vi "WSVCAP SHL Host LL RFFE Read.vi"(0 "RFFE Data [DUT Ordered]":u8[][](array[numeric]) format="%02x", 1 "Wait Ticks":u32, 2 "Slave Address":u8, 5 "Bytes to Read":u8, 7 "Socket Mask [U64]":u64=1 format="%02x", 11 "error in":errorcluster, 14 "FPGA":T1) -> (4 "RFFE Read Data [DUT Ordered]":u8[][](array[numeric]), 8 "Status":u8[](array[numeric]), 15 "error out":errorcluster)   [LabVIEW 2017]
uses:
  Type Defs/WSVCAP SHL FPGA Enum.ctl
  Type Defs/WSVCAP SHL Top Level Write Read State Enum.ctl
  Type Defs/WSVCAP SHL State.ctl
  Type Defs/WSVCAP SHL Top Level Control Enum.ctl
  Type Defs/WSVCAP SHL Transaction Enum.ctl
panel:
  out "Write Data":u64[](array[numeric]) format="%032b"
  out "Bit Array":u64[](array[numeric]) format="%.0x"
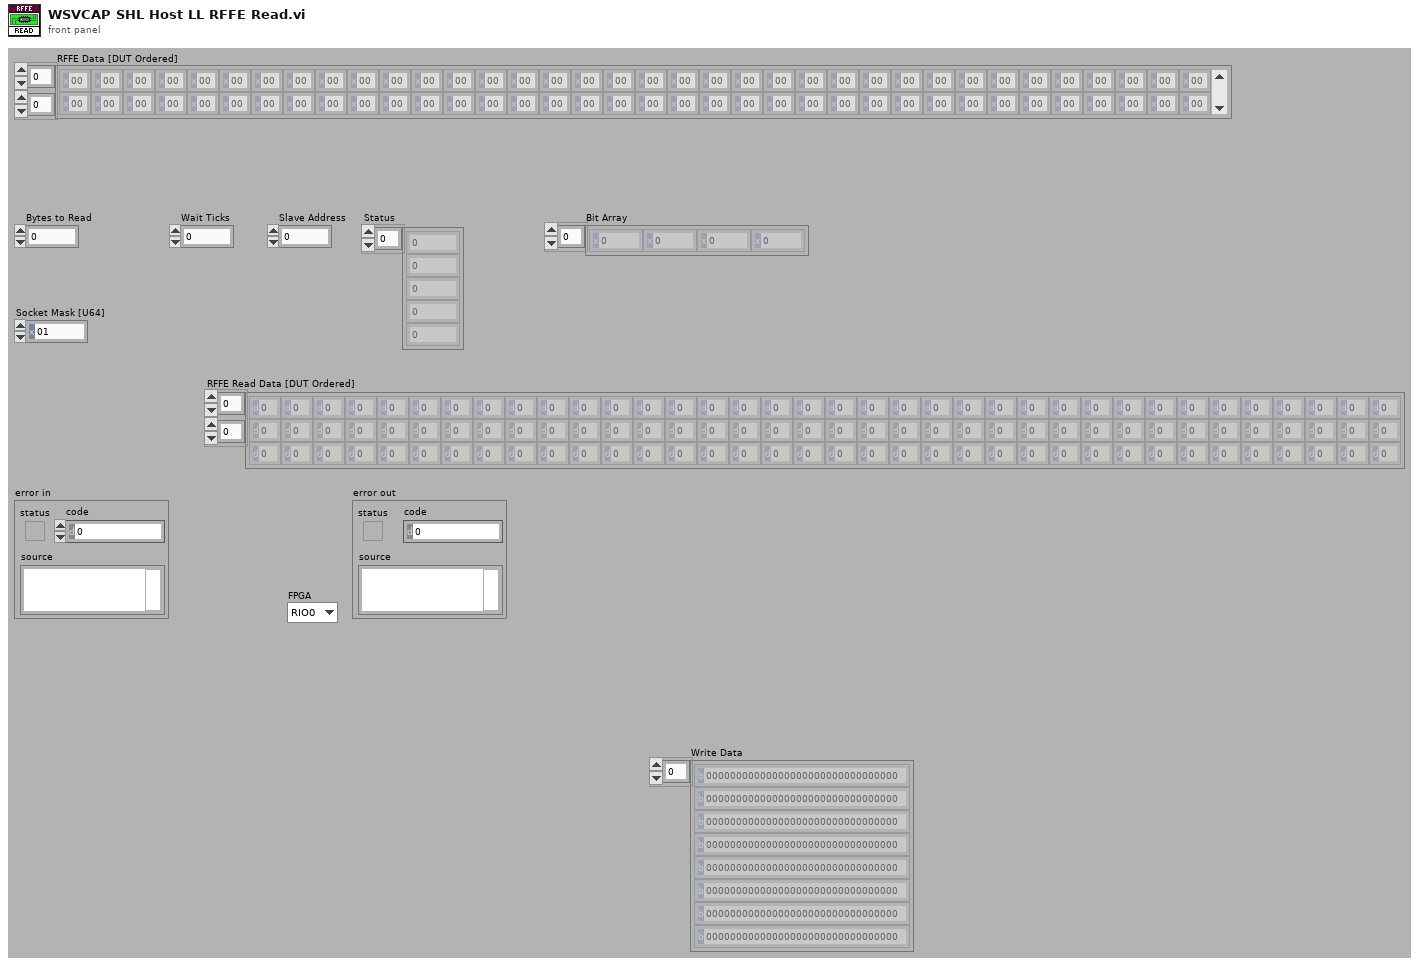
[diagram p1: front panel]
types:
  T1 = typedef "WSVCAP SHL FPGA Enum.ctl" = enum16{"RIO0", "RIO1"}
  T2 = typedef "WSVCAP SHL Top Level Write Read State Enum.ctl" = enum16{"Start", "Write", "Read", "Get Status", "Wait Until Done"}
  T3 = typedef "WSVCAP SHL State.ctl" = enum8{"Idle", "Transfer Data"}
  T4 = typedef "WSVCAP SHL Transaction Enum.ctl" = enum16{"I2C-Read Data", "I2C-Write Data", "RFFE-Ext Write", "RFFE-Ext Read"}
  T5 = typedef "WSVCAP SHL Top Level Control Enum.ctl" = enum16{"Start", "Cmd", "Transaction", "Wait Ticks", "Socket Mask", "UUT Set", "Slave Address", "Sub Address", "Bytes to Write", "Bytes to Read", "Write Data", "Write Flag", "Read Data", "Read Flag", "Ack Read", "Read Status Flag", "Ack Read Status", "Status", "Cycle Count", "Stop Cycle", "Exit"}
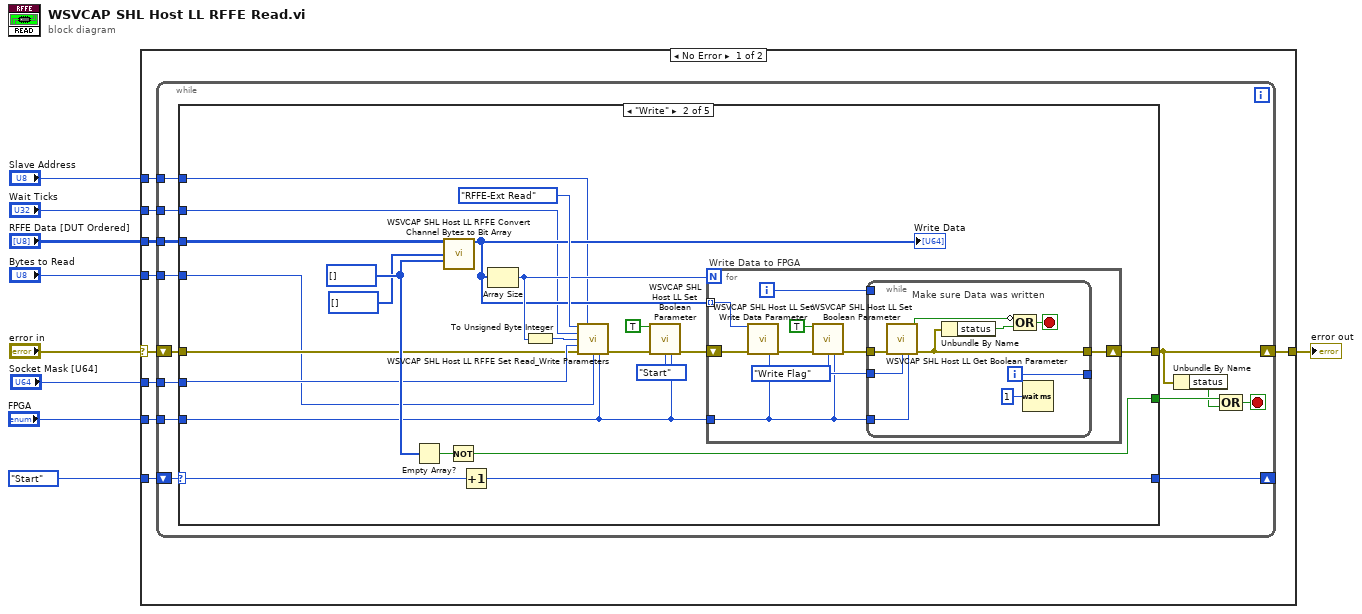
[diagram p0: block diagram]
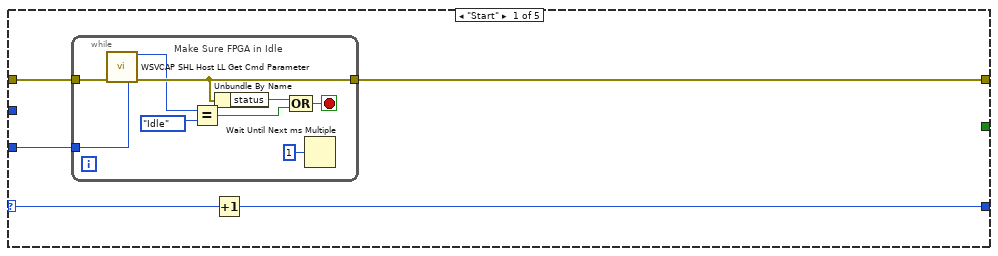
[diagram p2: hidden frame]
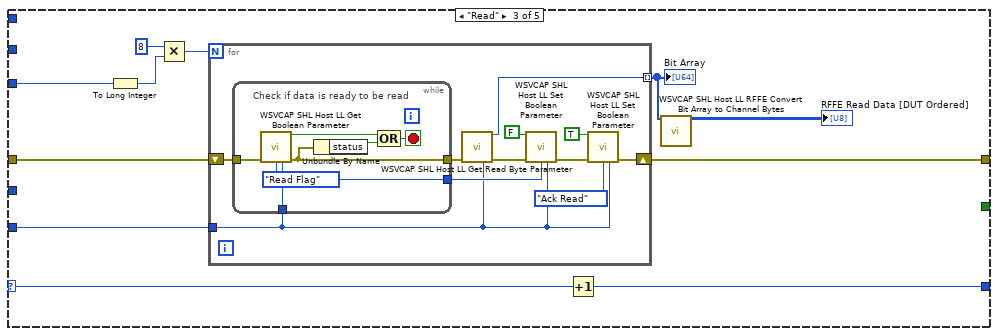
[diagram p3: hidden frame]
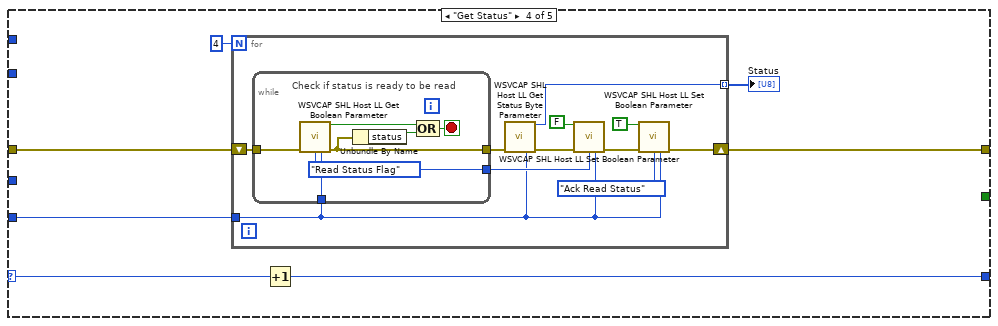
[diagram p4: hidden frame]
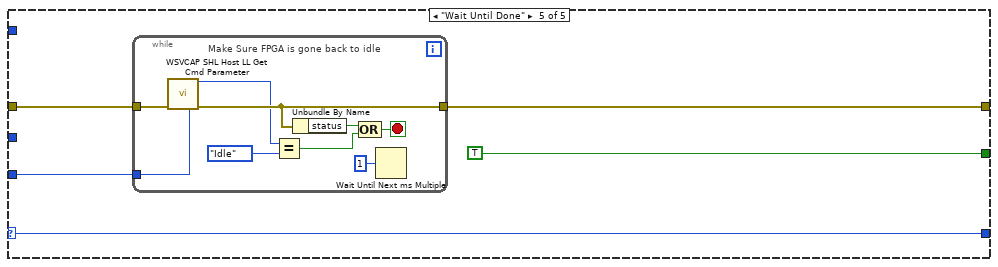
[diagram p5: hidden frame]
diagram:
  n1 = case shown="No Error" "error in" {
    selector: "error in" -> [w15 w154]
    tunnel: [w18 w154] -> w9
    tunnel: WSVCAP_SHL_Top_Level_Write_Read_State_Enum."Start" ("Write Read State") -> [w17 _]
    tunnel: "Socket Mask [U64]" -> [w16 _]
    tunnel: "Wait Ticks" -> [w14 _]
    tunnel: "Bytes to Read" -> [w13 _]
    tunnel: "Slave Address" -> [w12 _]
    tunnel: "RFFE Data [DUT Ordered]" -> [w11 _]
    tunnel: "FPGA" -> [w10 _]
    frame No Error {
      n2 = while {
        shift-right: [w30] -> w18
        shift-left: w15 -> [w31]
        shift-right: [w25] -> _
        shift-left: w17 -> [w26]
        tunnel: w16 -> [w24]
        tunnel: w14 -> [w23]
        tunnel: w13 -> [w22]
        tunnel: w12 -> [w21]
        tunnel: w11 -> [w20]
        tunnel: w10 -> [w19]
        stop <- w27 stop-if-true
        n3 = case shown="\"Write\"" w26 {
          selector: w26 -> [w35 w57 w96 w119 w142]
          tunnel: w31 -> [w36 w51 w90 w121 w144]
          tunnel: [w33 w55 w91 w120 w143] -> w30
          tunnel: [_ w48 _ _ TRUE] -> w29
          tunnel: [w34 w49 w95 w118 w142] -> w25
          tunnel: w24 -> [_ w56 _ _ _]
          tunnel: w23 -> [_ w52 _ _ _]
          tunnel: w22 -> [_ w47 w89 _ _]
          tunnel: w21 -> [_ w53 _ _ _]
          tunnel: w20 -> [_ w50 _ _ _]
          tunnel: w19 -> [w32 w46 w86 w115 w140]
          frame "Start" {
            n4 = while {
              tunnel: w36 -> [w41]
              tunnel: [w40] -> w33
              tunnel: w32 -> [w37]
              stop <- w45 stop-if-true
              # "Make Sure FPGA in Idle"
              n5 = call "WSVCAP SHL Host LL Get Cmd Parameter.vi"("error in (no error)"=w41, "FPGA"=w37) -> ("I2C_Cmd"=w39:T3, "error out"=w40:errorcluster)  [unwired: 12 in]
              n6 = Equal?(x=w39, y=WSVCAP_SHL_State."Idle" ("Type")) -> (x = y?=w43:bool)
              n7 = Unbundle By Name(w40) -> ("status"=w38:bool)
              n8 = Compound Arithmetic op=OR(w38, w43) -> (w45:bool)
              n9 = Wait Until Next ms Multiple(millisecond multiple=u32 1) -> ()  [unwired: 1 out]
            }
            n10 = Increment(x=w35) -> (x+1=w34:T2)
          }
          frame "Write" {
            w59 = u32[] [] ("Cycle CMD Delay Out (ticks)")
            # "Write Data to FPGA"
            n11 = Empty Array?(array=w59) -> (empty?=w60:bool)
            n12 = call "WSVCAP SHL Host LL RFFE Convert Channel Bytes to Bit Array.vi"("RFFE Data"=w50, "Cycle CMD Lengths Out (bits)"=u8[] [], "Cycle CMD Delay Out (ticks)"=w59) -> ("Write Data"=w58:u64[])  [unwired: 12 in]
            "Write Data" <- w58
            n13 = Not(x=w60) -> (.not. x?=w48:bool)
            n14 = Increment(x=w57) -> (x+1=w49:T2)
            n15 = Array Size(array=w58) -> (size(s)=w66:i32)
            n16 = To Unsigned Byte Integer(number=w66) -> (unsigned 8bit integer=w64:u8)
            n17 = call "WSVCAP SHL Host LL RFFE Set Read_Write Parameters.vi"("Transaction"=WSVCAP_SHL_Transaction_Enum."RFFE-Ext Read", "Slave Address"=w53, "Wait Ticks"=w52, "Bytes to Write"=w64, "Socket Mask [U64]"=w56, "error in (no error)"=w51, "Bytes to Read (Ext-Read Only)"=w47, "FPGA"=w46) -> ("error out"=w61:errorcluster)  [unwired: 7 in]
            n18 = call "WSVCAP SHL Host LL Set Boolean Parameter.vi"("Boolean In"=TRUE, "error in (no error)"=w61, "FPGA Top Level Control"=WSVCAP_SHL_Top_Level_Control_Enum."Start", "FPGA"=w46) -> ("error out"=w65:errorcluster)  [unwired: 11 in]
            n19 = for {
              N: w66 -> [_]
              shift-right: [w76] -> w55
              shift-left: w65 -> [w75]
              tunnel: w58 -> [w74] mode=indexing
              tunnel: w46 -> [w68]
              i -> [w69]
              w70 = WSVCAP_SHL_Top_Level_Control_Enum."Write Flag" ("FPGA Top Level Control")
              n20 = call "WSVCAP SHL Host LL Set Write Data Parameter.vi"("Write Byte In"=w74, "error in (no error)"=w75, "FPGA"=w68) -> ("error out"=w73:errorcluster)  [unwired: 12 in]
              n21 = call "WSVCAP SHL Host LL Set Boolean Parameter.vi"("Boolean In"=TRUE, "error in (no error)"=w73, "FPGA Top Level Control"=w70, "FPGA"=w68) -> ("error out"=w71:errorcluster)  [unwired: 11 in]
              n22 = while {
                tunnel: w71 -> [w83]
                tunnel: [w82] -> w76
                tunnel: w70 -> [w80]
                tunnel: w69 -> [_]
                tunnel: [w78] -> _
                tunnel: w68 -> [w77]
                i -> [w78]
                stop <- w85 stop-if-true
                # "Make sure Data was written"
                n23 = call "WSVCAP SHL Host LL Get Boolean Parameter.vi"("error in (no error)"=w83, "FPGA Top Level Control"=w80, "FPGA"=w77) -> ("Boolean Out"=w81:bool, "error out"=w82:errorcluster)  [unwired: 11 in]
                n24 = Unbundle By Name(w82) -> ("status"=w79:bool)
                n25 = Compound Arithmetic op=OR(invert w81, w79) -> (w85:bool)
                n26 = Wait (ms)(milliseconds to wait=u32 1) -> ()  [unwired: 1 out]
              }
            }
          }
          frame "Read" {
            n27 = To Long Integer(number=w89) -> (32bit integer=w87:i32)
            n28 = Multiply(x=8, y=w87) -> (x*y=w93:i32)
            n29 = for {
              N: w93 -> [_]
              shift-right: [w104] -> w91
              shift-left: w90 -> [w107]
              tunnel: [w98] -> w94 mode=indexing
              tunnel: w86 -> [w97]
              n30 = while {
                tunnel: w107 -> [w112]
                tunnel: [w111] -> w106
                tunnel: [w109] -> w103
                tunnel: w97 -> [w108]
                stop <- w114 stop-if-true
                w109 = WSVCAP_SHL_Top_Level_Control_Enum."Read Flag" ("FPGA Top Level Control")
                # "Check if data is ready to be read"
                n31 = call "WSVCAP SHL Host LL Get Boolean Parameter.vi"("error in (no error)"=w112, "FPGA Top Level Control"=w109, "FPGA"=w108) -> ("Boolean Out"=w113:bool, "error out"=w111:errorcluster)  [unwired: 11 in]
                n32 = Unbundle By Name(w111) -> ("status"=w110:bool)
                n33 = Compound Arithmetic op=OR(w113, w110) -> (w114:bool)
              }
              n34 = call "WSVCAP SHL Host LL Get Read Byte Parameter.vi"("error in (no error)"=w106, "FPGA"=w97) -> ("Read Data In"=w98:u64, "error out"=w105:errorcluster)  [unwired: 12 in]
              n35 = call "WSVCAP SHL Host LL Set Boolean Parameter.vi"("Boolean In"=FALSE ("Read Flag"), "error in (no error)"=w105, "FPGA Top Level Control"=w103, "FPGA"=w97) -> ("error out"=w99:errorcluster)  [unwired: 11 in]
              n36 = call "WSVCAP SHL Host LL Set Boolean Parameter.vi"("Boolean In"=TRUE ("Write Flag"), "error in (no error)"=w99, "FPGA Top Level Control"=WSVCAP_SHL_Top_Level_Control_Enum."Ack Read", "FPGA"=w97) -> ("error out"=w104:errorcluster)  [unwired: 11 in]
            }
            "Bit Array" <- w94
            n37 = Increment(x=w96) -> (x+1=w95:T2)
            n38 = call "WSVCAP SHL Host LL RFFE Convert Bit Array to Channel Bytes.vi"("Bit Array"=w94) -> ("RFFE Read Data [Socket Ordered]"=→"RFFE Read Data [DUT Ordered]":u8[][])  [unwired: 14 in]
          }
          frame "Get Status" {
            n39 = for {
              N: 4 -> [_]
              shift-right: [w131] -> w120
              shift-left: w121 -> [w132]
              tunnel: [w123] -> w116 mode=indexing
              tunnel: w115 -> [w122]
              n40 = while {
                tunnel: w132 -> [w137]
                tunnel: [w136] -> w130
                tunnel: [w134] -> w128
                tunnel: w122 -> [w133]
                stop <- w139 stop-if-true
                w134 = WSVCAP_SHL_Top_Level_Control_Enum."Read Status Flag" ("FPGA Top Level Control")
                # "Check if status is ready to be read"
                n41 = call "WSVCAP SHL Host LL Get Boolean Parameter.vi"("error in (no error)"=w137, "FPGA Top Level Control"=w134, "FPGA"=w133) -> ("Boolean Out"=w138:bool, "error out"=w136:errorcluster)  [unwired: 11 in]
                n42 = Unbundle By Name(w136) -> ("status"=w135:bool)
                n43 = Compound Arithmetic op=OR(w138, w135) -> (w139:bool)
              }
              n44 = call "WSVCAP SHL Host LL Get Status Byte Parameter.vi"("error in (no error)"=w130, "FPGA"=w122) -> ("I2C Status Byte"=w123:u8, "error out"=w129:errorcluster)  [unwired: 12 in]
              n45 = call "WSVCAP SHL Host LL Set Boolean Parameter.vi"("Boolean In"=FALSE ("Read Flag"), "error in (no error)"=w129, "FPGA Top Level Control"=w128, "FPGA"=w122) -> ("error out"=w124:errorcluster)  [unwired: 11 in]
              n46 = call "WSVCAP SHL Host LL Set Boolean Parameter.vi"("Boolean In"=TRUE ("Write Flag"), "error in (no error)"=w124, "FPGA Top Level Control"=WSVCAP_SHL_Top_Level_Control_Enum."Ack Read Status", "FPGA"=w122) -> ("error out"=w131:errorcluster)  [unwired: 11 in]
            }
            "Status" <- w116
            n47 = Increment(x=w119) -> (x+1=w118:T2)
          }
          frame "Wait Until Done" {
            n48 = while {
              tunnel: w144 -> [w148]
              tunnel: [w147] -> w143
              tunnel: w140 -> [w145]
              stop <- w150 stop-if-true
              # "Make Sure FPGA is gone back to idle"
              n49 = call "WSVCAP SHL Host LL Get Cmd Parameter.vi"("error in (no error)"=w148, "FPGA"=w145) -> ("I2C_Cmd"=w146:T3, "error out"=w147:errorcluster)  [unwired: 12 in]
              n50 = Equal?(x=w146, y=WSVCAP_SHL_State."Idle") -> (x = y?=w151:bool)
              n51 = Unbundle By Name(w147) -> ("status"=w152:bool)
              n52 = Compound Arithmetic op=OR(w152, w151) -> (w150:bool)
              n53 = Wait Until Next ms Multiple(millisecond multiple=u32 1) -> ()  [unwired: 1 out]
            }
          }
        }
        n54 = Unbundle By Name(w30) -> ("status"=w28:bool)
        n55 = Compound Arithmetic op=OR(w29, w28) -> (w27:bool)
      }
    }
    frame Error {
    }
  }
  "error out" <- w9
